vi "ConvertGoop3ToGoop4_CreateInPlacementNode.vi"(8 "error in (no error)":errorcluster, 11 "ViRefIn":refnum<vi>) -> (0 "error out":errorcluster, 3 "ViRefOut":refnum<vi>)   [LabVIEW 2012]
uses:
  <resource>/Framework/Providers/Open_GDS/ClassProviders/Common/ScriptingFunctions/Scripting_FollowWireDownStreams_StopCriteria.ctl
  <resource>/Framework/Providers/Open_GDS/ClassProviders/Common/ScriptingFunctions/Scripting_NodeInfo.ctl
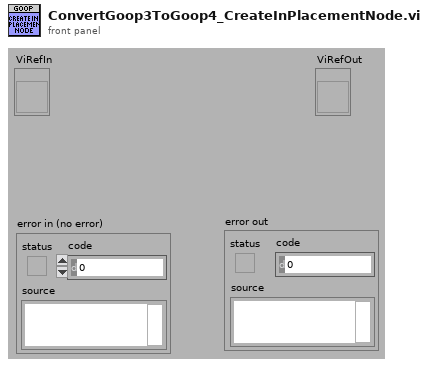
[diagram p1: front panel]
types:
  T1 = typedef "Scripting_FollowWireDownStreams_StopCriteria.ctl" = cluster{"ReachedANyOfTheseNodes":refnum<vi>[], "NodeType":string[], "VINames":string[], "AddTheseNodes":bool, "ALsoSerachOtherDrainNodes":bool}
  T2 = cluster{"Term Refnum Out":refnum<vi>, refnum<vi>[]}[]
  T3 = typedef "Scripting_NodeInfo.ctl" = cluster{"Type":string, "Style":string, "ObjectRef":refnum<vi>, "Terms":refnum<vi>[], "Sources":refnum<vi>[], "Drains":refnum<vi>[], "DrainsSourcesTerms":refnum<vi>[], "SourcesDrainTerms":cluster{"DrainsTerms":refnum<vi>[]}[], "UpperLeftPosition":cluster{"Left":i32, "Top":i32}, "LowerRightPosition":cluster{"Right":i32, "Bottom":i32}}
  T4 = typedef "LVPositionTypeDef.ctl" = cluster{"Left":i32, "Top":i32}
  T5 = typedef "LVBoundsTypeDef.ctl" = cluster{"Width":u32, "Height":u32}
  T6 = cluster{"Term Refnum Out":refnum<vi>, refnum<vi>[]}
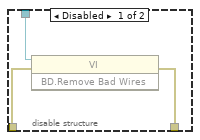
[diagram p2: hidden frame]
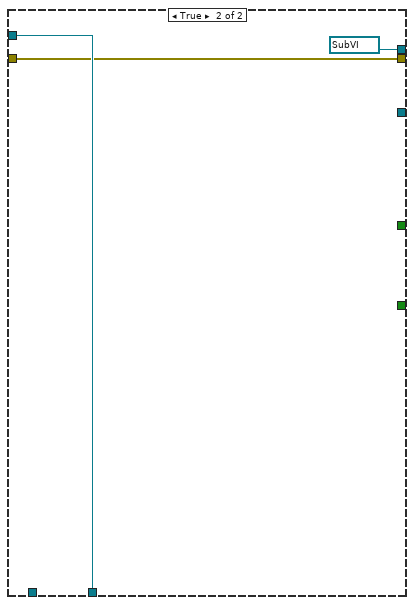
[diagram p5: hidden frame]
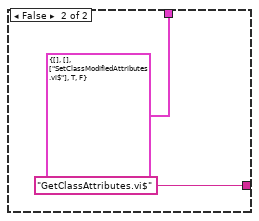
[diagram p7: hidden frame]
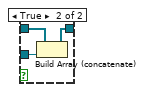
[diagram p11: hidden frame]
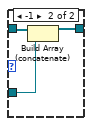
[diagram p12: hidden frame]
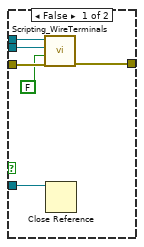
[diagram p15: hidden frame]
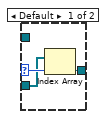
[diagram p19: hidden frame]
diagram:
  # "For every node\nGet all terms\nGet all sources\nGet all drains\nGet all sources drains\nget all drains sources"
  # "Get all nodes:\n-Along the 3 wires\n-All nodes between Get and Set"
  # "Find Get Attribute\nFollow the object wire until we get to the Set Attribute\n-All nodes passed will be inside the IPN\n-Check if there sources are constants and if so, are they inside to the left of GetA\n -For All UnBundler, check if one path leads to one of the Bundler, if so marks all object in that path"
  n1 = case shown="No Error" "error in (no error)" {
    selector: "error in (no error)" -> [w9 w627]
    tunnel: [w7 w627] -> w3
    tunnel: "ViRefIn" -> [w13 _]
    frame No Error {
      w4 = FALSE
      # "C:\\Projects\\GOOP3_To_GOOP4\\BaseSub\\Sub class\\SetClassAttribute.vi"
      n2 = property class="VI"(reference=w13, error in=w9) -> (reference out=w5:refnum<vi>, error out=w14:errorcluster, "Name"=w12:string)
      n3 = Match Pattern(string=w12, regular expression="TP_XA173 WriteConfig.vi") -> (offset past match=w11:i32)  [unwired: 1 in, 3 out]
      n4 = Greater Or Equal To 0?(x=w11) -> ()  [unwired: 1 out]
      n5 = property class="VI"(reference=w5, error in=w14, "BDWin.Open"=w4) -> (error out=w17:errorcluster)  [unwired: 1 out]
      n6 = case shown="True" w4 {
        frame False {
        }
        frame True {
        }
      }
      n7 = call <resource>:"Scripting_FindNodeOnDiagram_1.vi"("ViRef(Ignored If Not Wired)"=w5, "NodeTypesToSearchFor"=string[] ["SubVI"], "error in (no error)"=w17) -> ("Nodes"=w18:refnum<vi>[], "error out"=w19:errorcluster)  [unwired: 15 in]
      n8 = for {
        tunnel: w18 -> [w29] mode=indexing
        shift-right: [w27] -> w8
        shift-left: w19 -> [w43]
        tunnel: w5 -> [w39]
        shift-right: [w32] -> w10
        shift-left: refnum<vi>[] [] -> [w31]
        tunnel: [w30] -> w15 mode=indexing
        tunnel: w5 -> [w25]
        n9 = Not A Number/Path/Refnum?(number/path/refnum=w29) -> (NaN/Path/Refnum?=w28:bool)
        n10 = case shown="False" w28 {
          tunnel: w43 -> [w54 w81]
          tunnel: [w52 refnum<vi> refnum ("WhileLoop")] -> w42
          tunnel: [w51 w81] -> w41
          tunnel: [w50 _] -> w40
          tunnel: [w49 _] -> w35
          tunnel: [w48 _] -> w34
          tunnel: w31 -> [w47 _]
          tunnel: [w45 w82] -> w30
          tunnel: w29 -> [w44 w82]
          frame False {
            n11 = To More Specific Class(target class=refnum<vi> refnum ("WhileLoop"), reference=w44, error in=w54) -> (specific class reference=w45:refnum<vi>, error out=w53:errorcluster)
            n12 = Search 1D Array(1D array=w47, element=w45) -> (index of element=w46:i32)  [unwired: 1 in]
            n13 = case shown="-1" w46 {
              tunnel: w53 -> [w56 w79]
              tunnel: [w57 w77] -> w52
              tunnel: [w56 w76] -> w51
              tunnel: [_ w75] -> w50
              tunnel: [_ w60] -> w49
              tunnel: [_ w59] -> w48
              tunnel: w45 -> [w57 w58]
              frame 0, Default {
                # "It has already been deleted"
              }
              frame -1 {
                n14 = property class="SubVI"(reference=w58, error in=w79) -> (reference out=w77:refnum<vi>, error out=w76:errorcluster, "VIName"=w63:string, "Owner"=w75:refnum<vi>, "Desc"=w62:string)
                n15 = Match Pattern(string=w62, regular expression="M\\[[0-9]+:[0-9]+\\]") -> (offset past match=w72:i32)  [unwired: 1 in, 3 out]
                n16 = Match Pattern(string=w62, regular expression="CM\\[[0-9]+:[0-9]+\\]") -> (offset past match=w67:i32)  [unwired: 1 in, 3 out]
                n17 = Match Pattern(string=w63, regular expression="GetAttributes.vi$") -> (offset past match=w73:i32)  [unwired: 1 in, 3 out]
                n18 = Match Pattern(string=w63, regular expression="GetClassAttributes.vi$") -> (offset past match=w66:i32)  [unwired: 1 in, 3 out]
                n19 = Greater Or Equal To 0?(x=w72) -> (x >= 0?=w70:bool)
                n20 = Greater Or Equal To 0?(x=w67) -> (x >= 0?=w69:bool)
                n21 = Greater Or Equal To 0?(x=w73) -> (x >= 0?=w71:bool)
                n22 = Greater Or Equal To 0?(x=w66) -> (x >= 0?=w68:bool)
                n23 = And(x=w71, y=w70) -> (x .and. y?=w59:bool)
                n24 = And(x=w68, y=w69) -> (x .and. y?=w61:bool)
                n25 = Or(x=w59, y=w61) -> (x .or. y?=w60:bool)
              }
            }
          }
          frame True {
          }
        }
        n26 = case shown="True" w35 {
          tunnel: w42 -> [w119 _]
          tunnel: w41 -> [w121 w626]
          tunnel: [w92 w626] -> w27
          tunnel: w40 -> [w112 _]
          tunnel: w39 -> [w85 _]
          tunnel: [w106 _] -> w38
          tunnel: [w101 _] -> w37
          tunnel: [w100 _] -> w36
          tunnel: w34 -> [w98 _]
          tunnel: [w95 _] -> w33
          tunnel: [w94 w625] -> w32
          tunnel: w31 -> [w93 w625]
          tunnel: [w86 _] -> w26
          tunnel: w25 -> [w84 _]
          frame True {
            # "All Get Att Drains\n(Left Terminals)"
            # "ErrorOut"
            # "Att"
            # "ErrorOut"
            # "Att"
            n27 = property class="SubVI"(reference=w119, error in=w121) -> (reference out=w111:refnum<vi>, error out=w118:errorcluster, "Terms[]"=w89:refnum<vi>[])
            n28 = call <resource>:"Scripting_SortTerminals.vi"("Terminals[]"=w89) -> ("TerminalsOut[]"=w83:refnum<vi>[])  [unwired: 8 in, 2 out]
            n29 = Array Size(array=w89) -> (size(s)=w122:i32)
            n30 = case shown="True" w98 {
              tunnel: [T1 {"ReachedANyOfTheseNodes"=[], "NodeType"=[], "VINames"=["SetModifiedAttributes.vi$"], "AddTheseNodes"=TRUE, "ALsoSerachOtherDrainNodes"=FALSE} ("StopCriteria") T1 {"ReachedANyOfTheseNodes"=[], "NodeType"=[], "VINames"=["SetClassModifiedAttributes.vi$"], "AddTheseNodes"=TRUE, "ALsoSerachOtherDrainNodes"=FALSE} ("StopCriteria")] -> w97
              tunnel: ["GetAttributes.vi$" ("regular expression") "GetClassAttributes.vi$" ("regular expression")] -> w96
              frame True {
              }
              frame False {
              }
            }
            n31 = for {
              tunnel: w89 -> [w130] mode=indexing
              shift-right: [w127] -> w87
              shift-left: refnum<vi>[] [] -> [w128]
              n32 = property class="Term"(reference=w130) -> (reference out=w129:refnum<vi>, "IsSource"=w126:bool, "Wire"=w123:refnum<vi>)  [unwired: 1 in, 1 out]
              n33 = Not A Number/Path/Refnum?(number/path/refnum=w123) -> (NaN/Path/Refnum?=w125:bool)
              n34 = Compound Arithmetic op=AND(w126, invert w125) -> (w124:bool)
              n35 = case shown="False" w124 {
                tunnel: w129 -> [w133 _]
                tunnel: w128 -> [w132 w134]
                tunnel: [w131 w134] -> w127
                frame False {
                  n36 = Build Array (concatenate)(w132, w133) -> (w131:refnum<vi>[])
                }
                frame True {
                }
              }
              n37 = Close Reference(reference=w123) -> ()  [unwired: 1 in, 1 out]
            }
            n38 = case shown="20" w122 {
              tunnel: [9 ("index") 15 ("index")] -> w104
              tunnel: [8 ("index") 14 ("index")] -> w103
              tunnel: [11 ("index") 19 ("index")] -> w105
              tunnel: [10 ("index") 17 ("index")] -> w102
              tunnel: [1 ("index") 2 ("index")] -> w90
              frame 12, Default {
              }
              frame 20 {
              }
            }
            n39 = Index Array(array=w83, index #1=w105, index #2=w104, index #3=w103, index #4=w102) -> (element #1=w114:refnum<vi>, element #2=w120:refnum<vi>, element #3=w117:refnum<vi>, element #4=w108:refnum<vi>)
            n40 = call <resource>:"Scripting_FollowWireDownStreams.vi"("Term Refnum"=w117, "NodeTypesToFind"=string[] ["SubVI"] ("NodeTypesToSearchFor"), "error in"=w118, "MainitainDataType"=TRUE ("MainitainDateType(True)"), "StopCriteria"=w97) -> ("Nodes"=w106:refnum<vi>[], "error out"=w109:errorcluster)  [unwired: 11 in, 2 out]
            n41 = Array Size(array=w106) -> (size(s)=w115:i32)
            n42 = Delete From Array(array=w106) -> (deleted portion=w113:refnum<vi>, array with subset deleted=w107:refnum<vi>[])  [unwired: 2 in]
            n43 = case shown="1.." w115 {
              tunnel: w120 -> [_ w219]
              tunnel: w114 -> [_ _]
              tunnel: w113 -> [_ w237]
              tunnel: w112 -> [_ w230]
              tunnel: w111 -> [_ w155]
              tunnel: [w140 w142] -> w110
              tunnel: w109 -> [w140 w148]
              tunnel: w108 -> [_ w208]
              tunnel: w90 -> [_ w223]
              tunnel: w107 -> [_ w220]
              tunnel: w105 -> [_ w146]
              tunnel: w104 -> [_ w218]
              tunnel: w103 -> [_ w217]
              tunnel: w102 -> [_ w216]
              tunnel: [_ w215] -> w101
              tunnel: [_ w214] -> w100
              tunnel: w85 -> [_ w165]
              tunnel: w96 -> [_ w191]
              tunnel: [_ w178] -> w95
              tunnel: [w139 w176] -> w94
              tunnel: w93 -> [w139 w175]
              tunnel: [_ w159] -> w91
              tunnel: w87 -> [_ w156]
              tunnel: [_ w151] -> w86
              tunnel: w84 -> [_ w149]
              tunnel: w83 -> [_ w147]
              frame 0, Default {
                # "We can't find the SetModifyVI, something is wrong"
              }
              frame 1.. {
                (unwired) refnum<vi> refnum ("element")
                w193 = refnum<vi>[] []
                w234 = refnum<vi> refnum  # InPlaceElementStructure
                w235 = 2360 items=[".NET Container"=2125, ".NET Refnum"=3441, "2D Picture"=3508, "3D Picture"=23776, "Absolute Value"=1054, "Access Rights"=1412, "ActiveX Container"=2072, "Add"=3915, "Add 1"=1050, "Add Array Elements"=1903, "Agitator"=3831, "AllSpoll"=1960, "Always Copy"=2400, "And"=1061, "And Array Elements"=1911, "Append True/False String"=1511, "Application Refnum"=3412, "Array"=21608, "Array 1"=3300, "Array Constant"=2070, "Array Interface Control"=23777, "Array Max & Min"=1907, "Array Size"=1809, "Array Subset"=2044, "Array To Cluster"=1168, "Array To Spreadsheet String"=1540, "Array of Strings to Path"=1422, "Atmospheric Tank"=3070, "Atmospheric Tank 1"=21751, "Automation Close"=8001, "Automation Open"=8000, "Automation Refnum"=3410, "Avogadro Constant (1/mol)"=23520, "Base 10 Logarithm Of e"=23512, "Bin"=3073, "Bin 1"=21755, "Bitpack to Array"=3135, "Blocking Variable Read"=23786, "Blocking Variable Write"=23789, "Bluetooth Close Connection"=9148, "Bluetooth Create Listener"=9151, "Bluetooth Discover"=9152, "Bluetooth Network Connection Refnum"=3468, "Bluetooth Open Connection"=9153, "Bluetooth Read"=9149, "Bluetooth Wait On Listener"=9147, "Bluetooth Write"=9150, "Boolean Array To Number"=1815, "Boolean To (0,1)"=1167, "Build Array"=2041, "Build Cluster Array"=2047, "Build Matrix"=8500, "Build Path"=1419, "Build Waveform"=2066, "Bundle"=2049, "Bundle By Name"=2057, "Byte Array To String"=1609, "Byte Stream File Refnum"=3408, "CAN Channel"=21966, "CAN Channel 1"=3340, "CAN Channel 2"=2124, "CAN Channel 3"=21817, "CAN Interface"=3339, "CAN Interface 1"=21815, "CAN Interface 2"=2123, "CAN Interface 3"=21964, "CAN Task"=3470, "CAN Task 1"=3471, "CAN Task 2"=21963, "CAN Task 3"=21789, "CPU Information"=24130, "Call By Reference Node"=3901, "Call Chain"=1999, "Call Library Function Node"=2062, "Call Parent Method"=2354, "Cancel Button"=21739, "Cancel Notification"=9107, "Carriage Return Constant"=23500, "Case Structure"=2001, "Cast Unit Bases"=1079, "Check Valve"=3833, "Checkbox"=3117, "Class Specifier Constant"=2094, "Classic Radio Buttons"=22003, "Clear Fixed-Point Overflow Status"=5562, "Close File"=1405, "Close File 1"=8052, "Close Reference"=8011, "Close Variable Connection"=23783, "Cluster"=3400, "Cluster 1"=21607, "Cluster Constant"=2071, "Cluster To Array"=1169, "Code Interface Node"=2050, "Coerce To Type"=2402, "Color Box"=3013, "Color Box Constant"=2120, "Color Box Thin Border"=2905, "Color Ramp"=3022, "Combo Box"=21604, "Combo Box 1"=3304, "Combo Box Constant"=2088, "Complex Conjugate"=1048, "Complex To Polar"=1045, "Complex To Re/Im"=1044, "Compound Arithmetic"=2200, "Compressor"=3832, "Concatenate Strings"=2040, "Conditional Disable Structure"=2064, "Constructor Node"=3904, "Control & Simulation Loop"=2099, "Control Help Window"=1353, "Control Online Help"=1355, "Control Refnum"=3419, "Convert Unit"=2059, "Conveyer"=3827, "Copy"=1416, "Copy 1"=8053, "Cosecant"=1204, "Cosine"=1201, "Cotangent"=1205, "Create Folder"=8055, "Create User Event"=2073, "Current Processor ID"=24131, "Current VI's Menubar"=9000, "Current VI's Path"=1426, "DAQmx Analog Trigger Source"=3336, "DAQmx Analog Trigger Source 1"=2119, "DAQmx Analog Trigger Source 2"=21951, "DAQmx Analog Trigger Source 3"=21774, "DAQmx Device Name"=21773, "DAQmx Device Name 1"=21950, "DAQmx Device Name 2"=2093, "DAQmx Device Name 3"=3318, "DAQmx Global Channel"=3443, "DAQmx Global Channel 1"=21770, "DAQmx Global Channel 2"=21957, "DAQmx Global Channel 3"=3430, "DAQmx Physical Channel"=3335, "DAQmx Physical Channel 1"=21954, "DAQmx Physical Channel 2"=2118, "DAQmx Physical Channel 3"=21777, "DAQmx Scale Name"=21952, "DAQmx Scale Name 1"=21775, "DAQmx Scale Name 2"=3317, "DAQmx Scale Name 3"=2116, "DAQmx Switch"=21953, "DAQmx Switch 1"=3337, "DAQmx Switch 2"=2121, "DAQmx Switch 3"=21776, "DAQmx Task Name"=3442, "DAQmx Task Name 1"=3434, "DAQmx Task Name 2"=21959, "DAQmx Task Name 3"=21778, "DAQmx Terminal"=21955, "DAQmx Terminal 1"=2117, "DAQmx Terminal 2"=21781, "DAQmx Terminal 3"=3319, "Data Cache Size"=24132, "Data Log File Refnum"=3402, "DataSocket Close"=1085, "DataSocket Open"=1084, "DataSocket Read"=1086, "DataSocket Refnum"=3417, "DataSocket Write"=1087, "Date/Time To Seconds"=1308, "Decimal Digit?"=1119, "Decimal String To Number"=1184, "Decimate 1D Array"=2046, "DecomposeArray"=2412, "DecomposeLockDataValRef"=2406, "DecomposeVariant"=2404, "Decrement"=1058, "Default Directory"=1427, "Delete"=8056, "Delete 1"=1417, "Delete Data Value Reference"=2409, "Delete From Array"=3912, "Delete Menu Items"=9004, "Delete Variant Attribute"=8206, "Delete Waveform Attribute"=8209, "Deny Access"=8057, "Dequeue Element"=9113, "Destroy User Event"=2075, "DevClear"=1961, "DevClearList"=1962, "Device Control/Status"=1433, "Device Refnum"=3405, "Diagram Disable Structure"=2054, "Dial"=3050, "Dial 1"=21732, "Digital Data"=3210, "Digital Data 1"=21216, "Digital Waveform Graph"=21718, "Digital Waveform Graph 1"=3511, "Direct Variable Read"=23785, "Direct Variable Write"=23788, "Divide"=1053, "Divide 1"=3918, "Dlg CheckBox"=21924, "Dlg Horiz Scrollbar"=21905, "Dlg Numeric"=2100, "Dlg Numeric 2"=3006, "Dlg String"=2110, "Dlg Vert Scrollbar"=21906, "Down Arrow"=3824, "Down Bow Valve"=3707, "Down Bow Valve 1"=21767, "Down Bow Valve 2"=3807, "Down Rect Valve"=21766, "Down Rect Valve 1"=3706, "Down Rect Valve 2"=3806, "Down Tee"=3818, "Down Tee 1"=3718, "EOF"=1410, "Elementary Charge (C)"=23517, "Empty Array?"=23063, "Empty Path Constant"=23523, "Empty String Constant"=23503, "Empty String/Path?"=1112, "Enable Menu Tracking"=9002, "EnableLocal"=1963, "EnableRemote"=1964, "End of Line Constant"=23525, "Enqueue Element"=9111, "Enqueue Element At Opposite End"=9129, "Enum"=3023, "Enum 1"=21605, "Enum Constant"=2090, "Equal To 0?"=1113, "Equal?"=1102, "Error Ring Constant"=2039, "Event Callback Refnum"=3435, "Event Data Node"=2102, "Event Structure"=2052, "Exchanger"=3828, "Exclusive Or"=1063, "Exponential"=1211, "Exponential (Arg) -1"=1222, "Expression Node"=2201, "FIFO Refnum"=3474, "False Constant"=2006, "Feedback Node, Feedback Node 1"=2353, "FieldPoint IO Point"=21784, "FieldPoint IO Point 1"=3440, "FieldPoint IO Point 2"=3439, "File Dialog"=8058, "File Dialog 1"=8081, "File Path Control"=21730, "File Path Control 1"=3203, "File Path Indicator"=21731, "File Path Indicator 1"=3204, "File/Directory Info"=1413, "File/Directory Info 1"=8082, "FindLstn"=1965, "FindRQS"=1966, "First Call?"=1083, "Fixed-Point Overflow?"=5565, "Fixed-Point to Integer Cast"=5566, "Flat Box"=3602, "Flat Circle"=3605, "Flat Down Triangle"=3623, "Flat Frame"=3608, "Flat Left Triangle"=3620, "Flat Right Triangle"=3621, "Flat Round Button"=3102, "Flat Rounded Box"=3611, "Flat Sequence Structure"=2069, "Flat Square Button"=3103, "Flat Up Triangle"=3622, "Flatten To String"=1164, "Flatten To XML"=8400, "Flattened String To Variant"=8202, "Floating Point Equal?"=23064, "Flush File"=8059, "Flush File 1"=1406, "Flush Queue"=9114, "For Loop"=2002, "Fork"=2194, "Format Date/Time String"=8100, "Format Into File"=2083, "Format Into String"=2081, "Format Value"=1512, "Formula Node"=2004, "Fract/Exp String To Number"=1187, "Framed Color Box"=21019, "Framed Color Box 1"=3008, "Free Label"=2321, "Furnace"=3829, "GPIB Clear"=1954, "GPIB Initialization"=1957, "GPIB Misc"=1956, "GPIB Read"=1951, "GPIB Serial Poll"=1955, "GPIB Status"=1959, "GPIB Trigger"=1953, "GPIB Wait"=1958, "GPIB Write"=1950, "Gauge"=21009, "Gauge 1"=3040, "Generate Front Panel Activity"=1329, "Generate Occurrence"=1700, "Generate User Event"=2074, "Generate User-Defined Trace Event"=2250, "Get Datalog Position"=8061, "Get Date/Time In Seconds"=1303, "Get Date/Time String"=1600, "Get Drag Drop Data"=9154, "Get File Position"=8062, "Get File Size"=8063, "Get Fixed-Point Components"=11163, "Get Help Window Status"=1354, "Get Matrix Diagonal"=8501, "Get Matrix Elements"=8502, "Get Menu Item Info"=9005, "Get Menu Selection"=9001, "Get Menu Short Cut Info"=9007, "Get Notifier Status"=9103, "Get Number of Records"=8064, "Get Permissions"=8065, "Get Queue Status"=9110, "Get Submatrix"=8503, "Get Type and Creator"=8066, "Get Variant Attribute"=8205, "Get Volume Info"=8067, "Get Waveform Attribute"=8208, "Get Waveform Components"=2067, "Global Variable"=2060, "Gravitational Constant (N m2/kg2)"=23519, "Greater Or Equal To 0?"=1114, "Greater Or Equal?"=1103, "Greater Than 0?"=1117, "Greater?"=1110, "Handle Peek"=1604, "Handle Poke"=1605, "Hex Digit?"=1123, "Hexadecimal String To Number"=1185, "Hopper"=21754, "Hopper 1"=3072, "Horiz Line"=3821, "Horiz Pipe"=3710, "Horiz Pipe 1"=3810, "Horizontal Button Box"=3636, "Horizontal Fill Slide"=3012, "Horizontal Fill Slide 1"=21100, "Horizontal Graduated Bar"=21106, "Horizontal Pointer Slide"=21101, "Horizontal Pointer Slide 1"=3011, "Horizontal Progress Bar"=21102, "Horizontal Scrollbar"=21110, "Horizontal Slide"=3010, "Horizontal Slide Switch"=3114, "Horizontal Smooth Box"=3633, "Horizontal Splitter Bar"=21861, "Horizontal Splitter Bar (Classic)"=21863, "Horizontal Splitter Bar (System)"=21865, "Horizontal Switch"=3108, "Horizontal Tank"=3071, "Horizontal Toggle Switch"=3110, "Horizontal Toggle Switch 1"=21700, "Hyperbolic Cosecant"=23053, "Hyperbolic Cosine"=1215, "Hyperbolic Cotangent"=23055, "Hyperbolic Secant"=23054, "Hyperbolic Sine"=1214, "Hyperbolic Tangent"=1216, "IMAQ Session"=3415, "IP To String"=1710, "IVI Delete Session"=8103, "IVI Logical Name"=3420, "IVI Logical Name 1"=3414, "IVI Logical Name 2"=21736, "IVI New Session"=8102, "Implies"=1080, "In Place Element Structure"=2360, "In Range and Coerce"=1127, "Include Fixed-Point Overflow Status"=5564, "Increment"=1057, "Index & Bundle Cluster Array"=2056, "Index Array"=2042, "Index String Array"=1531, "Initialize Array"=2053, "Inline C Node"=2104, "Insert Into Array"=3911, "Insert Menu Items"=9003, "Integer to Fixed-Point Cast"=5567, "Intensity Chart"=21719, "Intensity Chart 1"=3509, "Intensity Graph"=21720, "Intensity Graph 1"=3510, "Interleave 1D Arrays"=2045, "Interpolate 1D Array"=1905, "Inverse Cosecant"=23050, "Inverse Cosine"=1207, "Inverse Cotangent"=23052, "Inverse Hyperbolic Cosecant"=23056, "Inverse Hyperbolic Cosine"=1218, "Inverse Hyperbolic Cotangent"=23058, "Inverse Hyperbolic Secant"=23057, "Inverse Hyperbolic Sine"=1217, "Inverse Hyperbolic Tangent"=1219, "Inverse Secant"=23051, "Inverse Sine"=1206, "Inverse Tangent"=1208, "Inverse Tangent (2 Input)"=1228, "Invoke Node"=3900, "IrDA Close Connection"=9144, "IrDA Create Listener"=9140, "IrDA Discover"=9141, "IrDA Network Connection Refnum"=3450, "IrDA Open Connection"=9142, "IrDA Read"=9145, "IrDA Wait On Listener"=9143, "IrDA Write"=9146, "Join"=2195, "Join Numbers"=1171, "Junction"=2197, "Knob"=21000, "Knob 1"=3005, "LED Button"=3116, "LabVIEW Object"=3457, "Label"=21960, "Labeled Oblong Button"=3125, "Labeled Rectangular Button"=3124, "Labeled Round Button"=3122, "Labeled Square Button"=3123, "Leak Variant Value Reference"=2410, "Left Arrow"=3826, "Left Bow Valve"=3701, "Left Bow Valve 1"=3801, "Left Bow Valve 2"=21761, "Left Down Elbow"=3711, "Left Down Elbow 1"=3811, "Left Pump"=3713, "Left Pump 1"=3813, "Left Rect Valve"=3700, "Left Rect Valve 1"=21760, "Left Rect Valve 2"=3800, "Left Tee"=3709, "Left Tee 1"=3809, "Left Up Elbow"=3808, "Left Up Elbow 1"=3708, "Less Or Equal To 0?"=1115, "Less Or Equal?"=1104, "Less Than 0?"=1118, "Less?"=1111, "Lexical Class"=1126, "Line Feed Constant"=23501, "List Directory"=1418, "List Folder"=8083, "Listbox"=21792, "Listbox 1"=21806, "Listbox Symbol Ring Constant"=2038, "Local Variable"=2061, "Lock Range"=1411, "Logarithm Base 10"=1210, "Logarithm Base 2"=1225, "Logarithm Base X"=1224, "Logical Shift"=1081, "Lossy Enqueue Element"=9130, "Lowered Rounded Box"=3638, "MATLAB script"=9020, "Machine Epsilon"=23528, "MakeAddr"=1967, "Mantissa & Exponent"=1150, "Match First String"=1532, "Match Pattern"=1535, "Match True/False String"=1533, "MathScript Call By Reference Node"=3906, "MathScript Node"=2357, "Matrix Size"=8507, "Max & Min"=1108, "Menu Refnum"=3413, "Menu Ring"=3018, "Menu Ring 1"=21600, "Menu-Popup Ring"=3017, "Merge Signals"=2350, "Meter"=21008, "Meter 1"=3030, "Mixed Signal Graph"=21721, "Molar Gas Constant (J/(mol K))"=23522, "Motion Resource"=21787, "Motion Resource 1"=3448, "Motion Resource 2"=3449, "Motor"=3720, "Motor 1"=3820, "Move"=1415, "Move 1"=8068, "Multi-Segment Pipe"=23780, "Multicolumn Listbox"=21799, "Multicolumn Listbox 1"=21791, "Multiple Selection Listbox"=3208, "Multiply"=1052, "Multiply 1"=3917, "Multiply Array Elements"=1904, "Multirate Structure"=2199, "Natural Logarithm"=1209, "Natural Logarithm (Arg +1)"=1221, "Natural Logarithm Base"=23510, "Natural Logarithm Of 10"=23513, "Natural Logarithm Of 2"=23514, "Natural Logarithm Of Pi"=23508, "Negate"=1069, "Negative Infinity"=23509, "New Data Value Reference"=2408, "New Directory"=1402, "New File"=1404, "New VI"=8014, "New VI Object"=8015, "Not"=1064, "Not A Number/Path/Refnum?"=1128, "Not A Path Constant"=23524, "Not And"=1071, "Not Equal To 0?"=1116, "Not Equal?"=1105, "Not Exclusive Or"=1073, "Not Or"=1072, "Not a Refnum Constant"=23526, "Not a Shared Variable"=23527, "Notifier Refnum"=3423, "Number To Boolean Array"=1814, "Number To Decimal String"=1180, "Number To Engineering String"=1183, "Number To Exponential String"=1505, "Number To Fractional String"=1506, "Number To Hexadecimal String"=1181, "Number To Octal String"=1182, "Number of Cache Levels"=24133, "Numeric Constant"=2005, "Numeric Control"=3000, "Numeric Control 1"=21003, "Numeric Indicator"=3001, "Numeric Indicator 1"=21004, "OK Button"=21738, "OLE Variant"=3150, "Obtain Notifier"=9101, "Obtain Queue"=9108, "Occurrence Refnum"=3406, "Octal Digit?"=1129, "Octal String To Number"=1186, "Old VISA Open"=1921, "One Button Dialog"=1340, "Open Application Reference"=8012, "Open Device"=1430, "Open File"=1403, "Open Tank"=21752, "Open Tank 1"=3074, "Open VI Object Reference"=8013, "Open VI Reference"=8010, "Open Variable Connection"=23779, "Open Variable Connection in Background"=23791, "Open and Verify Variable Connection"=23790, "Open/Create/Replace Datalog"=8054, "Open/Create/Replace File"=8050, "Or"=1062, "Or Array Elements"=1910, "PPoll"=1969, "PPollConfig"=1970, "PPollUnconfig"=1971, "Package Matrix"=23001, "PassControl"=1968, "Path Constant"=2009, "Path To String"=1077, "Path Type"=1421, "Path to Array of Strings"=1423, "Pi"=23504, "Pi Divided By 2"=23506, "Pi Multiplied By 2"=23505, "Pick Line"=1510, "Pict Ring"=21602, "Pict Ring 1"=3015, "PixMap"=3505, "PixMap (Do not touch it!!)"=3507, "Planck's Constant (J/Hz)"=23516, "Platform Flat Square Button"=3134, "Plug-In Control"=21820, "Polar To Complex"=1047, "Polar To Re/Im"=23061, "Positive Infinity"=23515, "Power Of 10"=1212, "Power Of 2"=1223, "Power Of X"=1213, "Preserve Run-Time Class"=8018, "Pressure Tank"=3075, "Pressure Tank 1"=21753, "Preview Queue Element"=9112, "Printable?"=1124, "Property Node"=1920, "Pulldown Menu Ring"=3061, "Push Button"=21001, "Queue Refnum"=3424, "Quit LabVIEW"=1352, "Quotient & Remainder"=1056, "RT FIFO Create"=24000, "RT FIFO Delete"=24003, "RT FIFO Read"=24001, "RT FIFO Write"=24002, "Radio Buttons"=22001, "Raised Box"=3600, "Raised Box 1"=3637, "Raised Circle"=3603, "Raised Down Triangle"=3615, "Raised Frame"=3606, "Raised Left Triangle"=3612, "Raised Right Triangle"=3613, "Raised Rounded Box"=3609, "Raised Up Triangle"=3614, "Random Number (0-1)"=1070, "RcvRespMsg"=1972, "Re/Im To Complex"=1046, "Re/Im To Polar"=23060, "Read Datalog"=8069, "Read Device"=1432, "Read File"=1407, "Read Variable"=23781, "Read from Binary File"=8051, "Read from Text File"=8070, "ReadStatus"=1973, "Receive"=1974, "ReceiveSetup"=1975, "Recessed Box"=3601, "Recessed Circle"=3604, "Recessed Down Triangle"=3619, "Recessed Frame"=3607, "Recessed Left Triangle"=3616, "Recessed Menu Ring"=3019, "Recessed Right Triangle"=3617, "Recessed Rounded Box"=3610, "Recessed Up Triangle"=3618, "Reciprocal"=1059, "Reciprocal Of Pi"=23507, "Reciprocal Of e"=23511, "RecomposeArray"=2403, "RecomposeUnlockDataValRef"=2407, "RecomposeVariant"=2405, "Rectangular Stop Button"=3128, "Refnum to Path"=1424, "Refnum to Session"=2306, "Region"=2196, "Register Event Callback"=2078, "Register For Events"=2065, "Register Session"=2319, "Release Notifier"=9102, "Release Queue"=9109, "Remove Fixed-Point Overflow Status"=5563, "Replace Array Subset"=3910, "Replace Substring"=3913, "Request Deallocation"=1610, "ResetSys"=1976, "Reshape Array"=2055, "Resize Matrix"=8508, "Reverse 1D Array"=1900, "Reverse String"=1537, "Right Arrow"=3825, "Right Bow Valve"=21765, "Right Bow Valve 1"=3705, "Right Bow Valve 2"=3805, "Right Down Elbow"=3817, "Right Down Elbow 1"=3717, "Right Pump"=3719, "Right Pump 1"=3819, "Right Rect Valve"=3804, "Right Rect Valve 1"=3704, "Right Rect Valve 2"=21764, "Right Tee"=3715, "Right Tee 1"=3815, "Right Up Elbow"=3814, "Right Up Elbow 1"=3714, "Ring Constant"=2008, "Rocker"=21002, "Rotary Feeder"=3830, "Rotate"=1082, "Rotate 1D Array"=1906, "Rotate Left With Carry"=1606, "Rotate Right With Carry"=1607, "Rotate String"=1536, "Round Button"=3100, "Round LED"=3120, "Round LED 1"=21012, "Round Light"=3104, "Round Push Button"=3112, "Round Push Button 2"=3118, "Round Radio Button"=3106, "Round Stop Button"=3127, "Round To Nearest"=1055, "Round Toward +Infinity"=1076, "Round Toward -Infinity"=1075, "Rydberg Constant (1/m)"=23521, "Scale By Power Of 2"=1074, "Scan From File"=2082, "Scan From String"=2080, "Scan String For Tokens"=8101, "Scan Value"=1534, "Scanned Variable Read"=23784, "Scanned Variable Write"=23787, "Search 1D Array"=1901, "Search and Replace String"=3914, "Search/Split String"=1538, "Secant"=1203, "Seconds To Date/Time"=1309, "Seek"=1409, "Select"=1516, "Send"=1977, "Send Notification"=9104, "SendCmds"=1978, "SendDataBytes"=1979, "SendIFC"=1980, "SendLLO"=1982, "SendList"=1981, "SendSetup"=1983, "Session to Refnum"=2307, "Set Datalog Position"=8072, "Set File Position"=8073, "Set File Size"=8074, "Set Matrix Diagonal"=8504, "Set Matrix Elements"=8505, "Set Menu Item Info"=9006, "Set Number of Records"=8075, "Set Occurrence"=1702, "Set Permissions"=8076, "Set Submatrix"=8506, "Set Type and Creator"=8077, "Set Variant Attribute"=8204, "Set Waveform Attribute"=8207, "SetRWLS"=1984, "SetTimeOut"=1985, "Shared Variable"=23778, "Shared Variable Constant"=3473, "Shared Variable Control"=3472, "Shared Variable Control 1"=21814, "Shared Variable to String"=1831, "Sign"=1049, "Simple Horizontal Slide"=3003, "Simple Numeric"=3029, "Simple Numeric 1"=2900, "Simple String"=2115, "Simple Vertical Slide"=3002, "Sinc"=1227, "Sine"=1200, "Sine & Cosine"=1220, "Size Handle"=1603, "Slide Switch"=21011, "Sort 1D Array"=1120, "Sort Array of String, Sort Array of String 1"=23065, "Speed Of Light In Vacuum (m/sec)"=23518, "Split 1D Array"=1908, "Split Button"=21020, "Split Number"=1170, "Split Signals"=2351, "Spreadsheet String To Array"=1539, "Square"=23059, "Square Button"=3101, "Square LED"=3121, "Square LED 1"=21013, "Square Light"=3105, "Square Push Button"=3113, "Square Push Button 2"=3119, "Square Radio Button"=3107, "Square Root"=1060, "Stacked Sequence Structure"=2000, "State"=2198, "State Diagram"=2051, "Static VI Reference"=2084, "Stop"=1350, "Stop Button"=21230, "String Constant"=2007, "String Control"=3200, "String Control 1"=21701, "String Indicator"=3201, "String Indicator 1"=21702, "String Length"=1502, "String Subset"=1503, "String To Byte Array"=1608, "String To IP"=1711, "String To Path"=1078, "String to Shared Variable"=1830, "Strip Path"=1420, "SubPanel"=21810, "SubPanel (Classic)"=21811, "SubPanel (System)"=21823, "Subtract"=1051, "Subtract 1"=3916, "Swap Bytes"=1162, "Swap Values"=2401, "Swap Vector Element"=1912, "Swap Words"=1163, "System Button"=3130, "System Cancel Button"=3131, "System Checkbox"=3132, "System Chiseled Line"=3632, "System Colored Rectangle"=3625, "System Combo Box"=21917, "System Enum"=3062, "System Horizontal Pointer Slide"=21902, "System Horizontal Progress Bar"=21910, "System Horizontal Slide"=21904, "System Label"=21961, "System Listbox"=21805, "System Mixed Checkbox"=21333, "System Multicolumn Listbox"=21798, "System Numeric"=21919, "System Path Control"=21922, "System Pict Ring"=21925, "System Radio Button"=3133, "System Radio Buttons"=22002, "System Recessed Frame"=3624, "System Ring"=3060, "System Spin Control"=21900, "System String"=21920, "System Tab Control"=3331, "System Table"=21797, "System Time Stamp"=21967, "System Tree"=21794, "System Vertical Pointer Slide"=21901, "System Vertical Progress Bar"=21909, "System Vertical Slide"=21903, "TCP Close Connection"=1713, "TCP Create Listener"=1717, "TCP Flattened Read"=1718, "TCP Flattened Write"=1719, "TCP Flex Read"=1720, "TCP Flex Write"=1721, "TCP Network Connection Refnum"=3407, "TCP Open Connection"=1715, "TCP Read"=1716, "TCP Wait On Listener"=1712, "TCP Write"=1714, "TDMS Close"=24113, "TDMS Defragment"=24119, "TDMS File"=3477, "TDMS Flush"=24117, "TDMS Get Properties"=24115, "TDMS List Contents"=24116, "TDMS Open"=24112, "TDMS Read"=24111, "TDMS Refnum To File ID"=24120, "TDMS Set Properties"=24114, "TDMS Write"=24110, "TDMS Write IP"=24118, "Tab Constant"=23502, "Tab Control"=3330, "Tab Control 1"=3332, "Table"=21796, "Table 1"=21790, "Tag Attribute Ring"=2063, "Tangent"=1202, "Tank"=21006, "Tank 1"=3020, "Temporary Directory"=1435, "TestSRQ"=1986, "TestSys"=1987, "Text & Pict Ring"=21603, "Text & Pict Ring 1"=3016, "Text Button"=21015, "Text Ring"=21601, "Text Ring 1"=3014, "Text to UTF-8"=23066, "Thermometer"=21007, "Thermometer 1"=3021, "Thick Chiseled Line"=3630, "Thick Line"=3629, "Thick Line with Arrow"=3631, "Thick Lowered Box"=3635, "Thin Chiseled Line"=3627, "Thin Line"=3626, "Thin Line with Arrow"=3628, "Threshold 1D Array"=1909, "Tick Count (ms)"=1300, "Time Stamp Constant"=2068, "Time Stamp Control"=21913, "Time Stamp Control 1"=5555, "Time Stamp Indicator"=21914, "Time Stamp Indicator 1"=5556, "Timed Loop"=5570, "Timed Sequence"=5573, "To Byte Integer"=1140, "To Double Precision Complex"=1152, "To Double Precision Float"=1147, "To Extended Precision Complex"=1154, "To Extended Precision Float"=1149, "To Fixed-Point"=5561, "To Long Integer"=1142, "To Lower Case"=1189, "To More Generic Class"=8017, "To More Specific Class"=8016, "To OLE Variant"=8002, "To Probe String"=2413, "To Quad Integer"=1155, "To Single Precision Complex"=1151, "To Single Precision Float"=1146, "To Time Stamp"=5560, "To Unsigned Byte Integer"=1143, "To Unsigned Long Integer"=1145, "To Unsigned Quad Integer"=1156, "To Unsigned Word Integer"=1144, "To Upper Case"=1188, "To Variant"=8201, "To Word Integer"=1141, "Traditional DAQ Channel"=21733, "Traditional DAQ Channel 1"=2085, "Traditional DAQ Channel 2"=3320, "Transpose 1D Array"=23068, "Transpose 2D Array"=1902, "Transpose Matrix"=8509, "Tree"=21819, "Tree 1"=21793, "Trigger"=1988, "TriggerList"=1989, "Two Button Dialog"=1341, "Type Cast"=1166, "Type and Creator"=1434, "UDP Close"=1726, "UDP Multicast Open"=1727, "UDP Network Connection Refnum"=3418, "UDP Open"=1723, "UDP Read"=1724, "UDP Write"=1725, "UTF-8 to Text"=23067, "Unbitpack from Array"=3136, "Unbundle"=2048, "Unbundle By Name"=2058, "Unflatten From String"=1165, "Unflatten From XML"=8401, "Unleak Variant Value Reference"=2411, "Unpackage Matrix"=23000, "Unregister For Events"=2076, "Unregister Session"=2320, "Up Arrow"=3823, "Up Bow Valve"=3703, "Up Bow Valve 1"=3803, "Up Bow Valve 2"=21763, "Up Rect Valve"=3702, "Up Rect Valve 1"=21762, "Up Rect Valve 2"=3802, "Up Tee"=3712, "Up Tee 1"=3812, "User Defined Refnum"=3428, "User Defined Refnum Tag"=21745, "User Defined Refnum Tag 1"=3429, "User Defined Refnum Tag Constant"=3426, "User Defined Refnum Tag Flatten"=21747, "User Defined Refnum Tag Flatten 1"=3454, "User Defined Tag"=21749, "User Defined Tag 1"=3329, "User Defined Tag Constant"=2114, "User Item"=3506, "VI Library"=1425, "VI Refnum"=3422, "VI Server Reference"=2091, "VISA Assert Interrupt Signal"=2309, "VISA Assert Trigger"=1929, "VISA Assert Utility Signal"=2310, "VISA Clear"=1927, "VISA Close"=1922, "VISA Disable Event"=1940, "VISA Discard Events"=1941, "VISA Enable Event"=1942, "VISA Find Resource"=1923, "VISA Flush I/O Buffer"=2302, "VISA GPIB Command"=2315, "VISA GPIB Control ATN"=2316, "VISA GPIB Control REN"=2304, "VISA GPIB Pass Control"=2317, "VISA GPIB Send IFC"=2318, "VISA In 16"=1930, "VISA In 32"=1944, "VISA In 64"=2140, "VISA In 8"=1936, "VISA Lock"=1993, "VISA Map Address"=1932, "VISA Map Trigger"=2311, "VISA Memory Allocation"=1997, "VISA Memory Allocation Ex"=2146, "VISA Memory Free"=1998, "VISA Move"=2303, "VISA Move In 16"=1948, "VISA Move In 32"=1991, "VISA Move In 64"=2144, "VISA Move In 8"=1946, "VISA Move Out 16"=1949, "VISA Move Out 32"=1992, "VISA Move Out 64"=2145, "VISA Move Out 8"=1947, "VISA Open"=2308, "VISA Out 16"=1931, "VISA Out 32"=1945, "VISA Out 64"=2141, "VISA Out 8"=1937, "VISA Peek 16"=1934, "VISA Peek 32"=1995, "VISA Peek 64"=2142, "VISA Peek 8"=1938, "VISA Poke 16"=1935, "VISA Poke 32"=1996, "VISA Poke 64"=2143, "VISA Poke 8"=1939, "VISA Read"=1925, "VISA Read STB"=1928, "VISA Read To File"=2313, "VISA Refnum to Session"=2300, "VISA Resource Name"=3421, "VISA Set I/O Buffer Size"=2301, "VISA Status Description"=1924, "VISA USB Control In"=2086, "VISA USB Control Out"=2087, "VISA Unlock"=1994, "VISA Unmap Address"=1933, "VISA Unmap Trigger"=2312, "VISA VXI Cmd or Query"=2305, "VISA Wait on Event"=1943, "VISA Write"=1926, "VISA Write From File"=2314, "VISA resource name"=3409, "VISA resource name 1"=21737, "Variable Class Specifier Constant"=2106, "Variable Configuration"=3475, "Variant"=3310, "Variant To Data"=8003, "Variant To Flattened String"=8203, "Vert Line"=3822, "Vert Pipe"=3816, "Vert Pipe 1"=3716, "Vert Rocker"=21740, "Vertical Fill Slide"=21014, "Vertical Fill Slide 1"=3009, "Vertical Graduated Bar"=21107, "Vertical Pointer Slide"=21017, "Vertical Pointer Slide 1"=3007, "Vertical Progress Bar"=21104, "Vertical Scrollbar"=21111, "Vertical Slide"=3004, "Vertical Slide Switch"=21741, "Vertical Slide Switch 1"=3115, "Vertical Smooth Box"=3634, "Vertical Splitter Bar"=21860, "Vertical Splitter Bar (Classic)"=21862, "Vertical Splitter Bar (System)"=21864, "Vertical Switch"=3109, "Vertical Toggle Switch"=21005, "Vertical Toggle Switch 1"=3111, "Volume Info"=1414, "Wait (ms)"=1302, "Wait For Activity"=1722, "Wait For Front Panel Activity"=1328, "Wait Until Next ms Multiple"=1327, "Wait for GPIB RQS"=1952, "Wait on Notification"=9105, "Wait on Notification from Multiple"=9106, "Wait on Notification from Multiple with Notifier History"=9132, "Wait on Notification with Notifier History"=9131, "Wait on Occurrence"=1701, "WaitSRQ"=1990, "Waveform Chart"=21010, "Waveform Chart 1"=3501, "Waveform Chart 2"=21717, "Waveform Graph"=21703, "Waveform Graph 1"=3504, "While Loop"=2003, "While Loop 1"=2352, "White Space?"=1125, "Write Datalog"=8079, "Write Device"=1431, "Write File"=1408, "Write Variable"=23782, "Write to Binary File"=8078, "Write to Text File"=8080, "XY Graph"=21716, "XY Graph 1"=3500, "Y-th Root of X"=23062]
                # "Get All Source\n(Right Terminals)"
                # "Get All nodes Drain Term Sources and get these Source Nodes\nAll drina terms.\nRemove the Drains terms that exists in the Nodes\nWe have in the array.\n==> Now we have some Source Nodes and their\nDrain Terminals that should be rewired are we're done"
                # "Last GetAtt ErrorOut"
                # "Last GetAtt ErrorOut"
                # "SetAtt Att Input Term"
                # "We need to add all nodes(SubVIs) between ErrorOut on last Get\nto the Error In of the SetAtt"
                # "Delete Wires to nodes"
                # "GetAtt No 1"
                # "GetAttToModifyForOtherlcassesIfNeeded"
                # "SetMod-VI"
                # "Rewire all nodes\nIf node when to GetAtt wire to DVR Inout Term\nIf node went to SetAtt wrie to DVR Out"
                # "DVR Ref"
                # "Remove Nodes that can be outside IPE"
                # "Get only Node Nodes"
                n44 = for {
                  tunnel: w220 -> [w587] mode=indexing
                  shift-right: [w574] -> w213
                  shift-left: w148 -> [w584]
                  tunnel: w146 -> [w578]
                  tunnel: w218 -> [w577]
                  tunnel: w217 -> [w576]
                  tunnel: w216 -> [w575]
                  shift-right: [w573] -> w214
                  shift-left: w193 -> [w572]
                  shift-right: [w571] -> w212
                  shift-left: w193 -> [w570]
                  shift-right: [w568] -> w206
                  shift-left: w193 -> [w569]
                  shift-right: [w566] -> w192
                  shift-left: w193 -> [w567]
                  tunnel: w191 -> [w565]
                  shift-right: [w564] -> w153
                  shift-left: w155 -> [w563]
                  # "GetAttSubVI"
                  n45 = To More Specific Class(target class=refnum<vi> refnum ("WhileLoop"), reference=w587, error in=w584) -> (specific class reference=w586:refnum<vi>, error out=w585:errorcluster)
                  n46 = property class="SubVI"(reference=w586, error in=w585) -> (reference out=w583:refnum<vi>, error out=w582:errorcluster, "VIName"=w581:string)
                  n47 = Match Pattern(string=w581, regular expression=w565) -> (offset past match=w580:i32)  [unwired: 1 in, 3 out]
                  n48 = Greater Or Equal To 0?(x=w580) -> (x >= 0?=w579:bool)
                  n49 = case shown="True" w579 {
                    tunnel: w583 -> [_ w614]
                    tunnel: w582 -> [w594 w613]
                    tunnel: w578 -> [_ w612]
                    tunnel: w577 -> [_ w611]
                    tunnel: w576 -> [_ w610]
                    tunnel: w575 -> [_ w609]
                    tunnel: [w594 w608] -> w574
                    tunnel: [w593 w607] -> w573
                    tunnel: w572 -> [w593 w606]
                    tunnel: [w592 w603] -> w571
                    tunnel: w570 -> [w592 w604]
                    tunnel: [w591 w601] -> w568
                    tunnel: w569 -> [w591 w600]
                    tunnel: [w590 w598] -> w566
                    tunnel: w567 -> [w590 w597]
                    tunnel: [w589 w595] -> w564
                    tunnel: w563 -> [w589 _]
                    frame False {
                    }
                    frame True {
                      n50 = property class="SubVI"(reference=w614, error in=w613) -> (reference out=w595:refnum<vi>, error out=w608:errorcluster, "Terms[]"=w605:refnum<vi>[])
                      n51 = Index Array(array=w605, index #1=w612, index #2=w611, index #3=w610, index #4=w609) -> (element #1=w596:refnum<vi>, element #2=w602:refnum<vi>, element #4=w599:refnum<vi>)  [unwired: 1 out]
                      n52 = Build Array (concatenate)(w606, w605) -> (w607:refnum<vi>[])
                      n53 = Build Array (concatenate)(w597, w596) -> (w598:refnum<vi>[])
                      n54 = Build Array (concatenate)(w604, w602) -> (w603:refnum<vi>[])
                      n55 = Build Array (concatenate)(w600, w599) -> (w601:refnum<vi>[])
                    }
                  }
                }
                n56 = To More Specific Class(target class=refnum<vi> refnum ("element"), reference=w237, error in=w213) -> (specific class reference=w177:refnum<vi>, error out=w231:errorcluster)
                n57 = property class="SubVI"(reference=w153) -> ("Terms[]"=w152:refnum<vi>[])  [unwired: 1 in, 2 out]
                n58 = for {
                  tunnel: w152 -> [w253] mode=indexing
                  shift-right: [w250] -> w151
                  shift-left: refnum<vi>[] [] -> [w251]
                  n59 = property class="Term"(reference=w253) -> (reference out=w252:refnum<vi>, "IsSource"=w249:bool, "Wire"=w246:refnum<vi>)  [unwired: 1 in, 1 out]
                  n60 = Not A Number/Path/Refnum?(number/path/refnum=w246) -> (NaN/Path/Refnum?=w248:bool)
                  n61 = Compound Arithmetic op=AND(w249, invert w248) -> (w247:bool)
                  n62 = case shown="False" w247 {
                    tunnel: w252 -> [w254 w258]
                    tunnel: w251 -> [w255 w257]
                    tunnel: [w255 w256] -> w250
                    frame False {
                      n63 = Close Reference(reference=w254) -> ()  [unwired: 1 in, 1 out]
                    }
                    frame True {
                      n64 = Build Array (concatenate)(w257, w258) -> (w256:refnum<vi>[])
                    }
                  }
                  n65 = Close Reference(reference=w246) -> ()  [unwired: 1 in, 1 out]
                }
                n66 = property class="SubVI"(reference=w177, error in=w231) -> (error out=w226:errorcluster, "Terms[]"=w215:refnum<vi>[])  [unwired: 1 out]
                n67 = call <resource>:"Scripting_SortTerminals.vi"("Terminals[]"=w215) -> ("TerminalsOut[]"=w224:refnum<vi>[])  [unwired: 8 in, 2 out]
                n68 = Build Array (concatenate)(w208, w206) -> (w207:refnum<vi>[])
                n69 = Index Array(array=w224, index=w223) -> (element=w160:refnum<vi>)
                n70 = Delete From Array(array=w192) -> (deleted portion=w180:refnum<vi>)  [unwired: 2 in, 1 out]
                n71 = Build Array (concatenate)(w219, w212) -> (w161:refnum<vi>[])
                n72 = for {
                  tunnel: [w526] -> w227 mode=indexing
                  tunnel: [w528] -> w221 mode=indexing
                  tunnel: w161 -> [w529] mode=indexing
                  shift-right: [w531] -> w225
                  shift-left: w226 -> [w532]
                  tunnel: [w525] -> w211 mode=indexing
                  tunnel: w160 -> [w523]
                  tunnel: T1 {"ReachedANyOfTheseNodes"=[], "NodeType"=[], "VINames"=["SetClassModifiedAttributes.vi$", "SetModifiedAttributes.vi$", "GetClassAttributes.vi$", "GetAttributes.vi$", "SetModifiedAttributes.vi$", "SetModifiedClassAttributes.vi$"], "AddTheseNodes"=FALSE, "ALsoSerachOtherDrainNodes"=FALSE} ("StopCriteria") -> [w514]
                  tunnel: w151 -> [_]
                  n73 = call <resource>:"Scripting_FollowWireDownStreams.vi"("Term Refnum"=w529, "NodeTypesToFind"=string[] ["NamedUnbundler", "NamedBundler"], "error in"=w532, "MainitainDataType"=TRUE ("MainitainDateType(True)"), "StopCriteria"=T1 {"ReachedANyOfTheseNodes"=[], "NodeType"=["SubVI", "PolymorphicSubVI", "CallParentNode", "DynamicDispatchSubVI"], "VINames"=[], "AddTheseNodes"=FALSE, "ALsoSerachOtherDrainNodes"=FALSE}) -> ("Nodes"=w519:refnum<vi>[], "NodeTypes"=w522:string[], "error out"=w533:errorcluster)  [unwired: 11 in, 1 out]
                  n74 = Reverse 1D Array(array=w522) -> (reversed array=w521:string[])
                  n75 = call <resource>:"Scripting_GetAllNodesConnectedToTerminal.vi"("Term Refnum"=w529, "error in"=w533, "StopCriteria"=w514) -> ("Nodes"=w535:refnum<vi>[], "error out"=w534:errorcluster)  [unwired: 13 in, 2 out]
                  n76 = Search 1D Array(1D array=w521, element="NamedBundler" ("regular expression")) -> (index of element=w517:i32)  [unwired: 1 in]
                  n77 = Reverse 1D Array(array=w519) -> (reversed array=w518:refnum<vi>[])
                  n78 = Index Array(array=w518, index=w517) -> (element=w516:refnum<vi>)
                  n79 = for {
                    tunnel: w535 -> [w538] mode=indexing
                    shift-right: [w543] -> w531
                    shift-left: w534 -> [w545]
                    shift-right: [w546] -> w527
                    shift-left: T3[] [] -> [w547]
                    tunnel: w523 -> [w540]
                    tunnel: w516 -> [w539]
                    n80 = call <resource>:"Scripting_GetNodeInfo.vi"("Node Refnum Or Constrol/Indicator/Constant"=w538, "error in (no error)"=w545) -> ("OK"=w544:bool, "NodeInfo"=w542:T3, "error out"=w543:errorcluster)  [unwired: 15 in]
                    n81 = Equal?(x=w538, y=w539) -> (x = y?=w537:bool)
                    n82 = case shown="True" w537 {
                      tunnel: w542 -> [w556 w558]
                      tunnel: [w557 w558] -> w541
                      tunnel: w540 -> [w548 _]
                      frame True {
                        w554 = 0 ("index")
                        n83 = Unbundle By Name(w556) -> ("SourcesDrainTerms"=w555:cluster{"DrainsTerms":refnum<vi>[]}[])
                        n84 = Index Array(array=w555, index=w554) -> (element=w552:cluster{"DrainsTerms":refnum<vi>[]})
                        n85 = Unbundle(w552) -> ("DrainsTerms"=w551:refnum<vi>[])
                        n86 = Build Array (concatenate)(w551, w548) -> (w550:refnum<vi>[])
                        n87 = Bundle(w550) -> (w549:cluster{refnum<vi>[]})  [unwired: 1 in]
                        n88 = Replace Array Subset(array=w555, new element=w549, index=w554) -> (w553:cluster{"DrainsTerms":refnum<vi>[]}[])
                        n89 = Bundle By Name(cluster=w556, "SourcesDrainTerms"=w553) -> (w557:T3)
                      }
                      frame False {
                      }
                    }
                    n90 = case shown="False" w544 {
                      tunnel: w547 -> [w559 w562]
                      tunnel: [w559 w561] -> w546
                      tunnel: w541 -> [_ w560]
                      frame False {
                      }
                      frame True {
                        n91 = Build Array (concatenate)(w562, w560) -> (w561:T3[])
                      }
                    }
                  }
                  n92 = Bundle("Nodes"=w519) -> (w525:cluster{"Nodes":refnum<vi>[]})  [unwired: 1 in]
                  n93 = Bundle("NodeTypes"=w522) -> (w528:cluster{"NodeTypes":string[]})  [unwired: 1 in]
                  n94 = Bundle(w527) -> (w526:cluster{T3[]})  [unwired: 1 in]
                }
                n95 = property class="Term"(reference=w180) -> ("Wire.Terms[]"=w178:refnum<vi>[])  [unwired: 1 in, 2 out]
                n96 = Search 1D Array(1D array=w178, element=w180) -> (index of element=w179:i32)  [unwired: 1 in]
                n97 = Delete From Array(array=w178, index=w179) -> ()  [unwired: 1 in, 2 out]
                n98 = call <resource>:"ConvertGoop3ToGoop4_SelectNodesToBeInsideIP.vi"("NodesIn"=w227, "BundleNodes"=w211, "BundleNodeTypes"=w221, "error in"=w225, "GetAttribute_AttributeTerminal"=w161, "FirstGetAttributesDrainsTerminals"=w156, "LastGetAttributesSourceTerminals"=w151) -> ("NodesOut"=w166:cluster{"NodesIn":T3[]}[], "IPE-Position"=w173:T4, "IPE-Frame Size"=w172:T5, "error out"=w171:errorcluster)  [unwired: 5 in]
                n99 = for {
                  tunnel: w166 -> [w284] mode=indexing
                  shift-right: [w285] -> w169
                  shift-left: refnum<vi>[] [] -> [w286]
                  n100 = Unbundle(w284) -> ("NodesIn"=w283:T3[])
                  n101 = for {
                    tunnel: w283 -> [w290] mode=indexing
                    shift-right: [w287] -> w285
                    shift-left: w286 -> [w288]
                    n102 = Unbundle By Name(w290) -> ("Drains"=w289:refnum<vi>[])
                    n103 = for {
                      tunnel: w289 -> [w292] mode=indexing
                      shift-right: [w291] -> w287
                      shift-left: w288 -> [w293]
                      n104 = Build Array (concatenate)(w293, w292) -> (w291:refnum<vi>[])
                    }
                  }
                }
                n105 = for {
                  tunnel: w166 -> [w298] mode=indexing
                  shift-right: [w299] -> w170
                  shift-left: w171 -> [w300]
                  tunnel: w169 -> [w296]
                  shift-right: [w294] -> w167
                  shift-left: T2 [] -> [w295]
                  n106 = Unbundle(w298) -> ("NodesIn"=w297:T3[])
                  n107 = for {
                    tunnel: w297 -> [w309] mode=indexing
                    shift-right: [w306] -> w299
                    shift-left: w300 -> [w307]
                    tunnel: w296 -> [w305]
                    shift-right: [w303] -> w294
                    shift-left: w295 -> [w301]
                    n108 = Unbundle By Name(w309) -> ("DrainsSourcesTerms"=w308:refnum<vi>[])  [unwired: 1 out]
                    n109 = for {
                      tunnel: w308 -> [w313] mode=indexing
                      shift-right: [w314] -> w306
                      shift-left: w307 -> [w316]
                      tunnel: w305 -> [w315]
                      shift-right: [w310] -> w304
                      shift-left: T2 [] -> [w311]
                      n110 = Not A Number/Path/Refnum?(number/path/refnum=w313) -> (NaN/Path/Refnum?=w312:bool)
                      n111 = case shown="False" w312 {
                        tunnel: w316 -> [w328 w339]
                        tunnel: w315 -> [w326 _]
                        tunnel: [w322 w339] -> w314
                        tunnel: w313 -> [w320 _]
                        tunnel: w311 -> [w318 w340]
                        tunnel: [w319 w340] -> w310
                        frame False {
                          n112 = call <resource>:"Scripting_GetTerminalWireConnectionPoints.vi"("Term Refnum In"=w320, "error in"=w328) -> ("Term Refnum Out"=w323:refnum<vi>, "WireTermSource"=w321:refnum<vi>, "AllWireTerminalDrains"=w327:refnum<vi>[], "error out"=w322:errorcluster)  [unwired: 9 in, 5 out]
                          n113 = Close Reference(reference=w321) -> ()  [unwired: 1 in, 1 out]
                          n114 = for {
                            tunnel: w327 -> [w331] mode=indexing
                            tunnel: w326 -> [w333]
                            shift-right: [w329] -> w324
                            shift-left: refnum<vi>[] [] -> [w330]
                            n115 = Search 1D Array(1D array=w333, element=w331) -> (index of element=w332:i32)  [unwired: 1 in]
                            n116 = case shown="0, Default" w332 {
                              tunnel: w331 -> [w335 w336]
                              tunnel: w330 -> [w334 w337]
                              tunnel: [w334 w338] -> w329
                              frame 0, Default {
                                n117 = Close Reference(reference=w335) -> ()  [unwired: 1 in, 1 out]
                              }
                              frame -1 {
                                n118 = Build Array (concatenate)(w337, w336) -> (w338:refnum<vi>[])
                              }
                            }
                          }
                          n119 = Bundle("Term Refnum Out"=w323, w324) -> (w317:T6)  [unwired: 1 in]
                          n120 = Build Array (concatenate)(w318, w317) -> (w319:T2)
                        }
                        frame True {
                        }
                      }
                    }
                    n121 = Build Array (concatenate)(w301, w304) -> (w303:T2)
                  }
                }
                n122 = for {
                  tunnel: w166 -> [w491] mode=indexing
                  shift-right: [w492] -> w222
                  shift-left: w170 -> [w493]
                  n123 = Unbundle(w491) -> ("NodesIn"=w490:T3[])
                  n124 = for {
                    tunnel: w490 -> [w497] mode=indexing
                    shift-right: [w494] -> w492
                    shift-left: w493 -> [w495]
                    n125 = Unbundle By Name(w497) -> ("Terms"=w496:refnum<vi>[])
                    n126 = for {
                      tunnel: w496 -> [w501] mode=indexing
                      shift-right: [w498] -> w494
                      shift-left: w495 -> [w502]
                      n127 = Not A Number/Path/Refnum?(number/path/refnum=w501) -> (NaN/Path/Refnum?=w500:bool)
                      n128 = case shown="False" w500 {
                        tunnel: w502 -> [w508 w513]
                        tunnel: [w505 w513] -> w499
                        tunnel: w501 -> [w503 _]
                        frame False {
                          n129 = property class="Term"(reference=w503, error in=w508) -> (error out=w507:errorcluster, "Wire"=w504:refnum<vi>)  [unwired: 1 out]
                          n130 = Not A Number/Path/Refnum?(number/path/refnum=w504) -> (NaN/Path/Refnum?=w506:bool)
                          n131 = case shown="False" w506 {
                            tunnel: w504 -> [w511 _]
                            tunnel: w507 -> [w510 w512]
                            tunnel: [w509 w512] -> w505
                            frame False {
                              n132 = invoke class="Wire" method="Delete"(reference=w511, error in=w510) -> (error out=w509:errorcluster)  [unwired: 1 in, 2 out]
                            }
                            frame True {
                            }
                          }
                        }
                        frame True {
                        }
                      }
                      n133 = call <vilib>:"Clear Errors.vi"("error in (no error)"=w499) -> ("error out"=w498:errorcluster)  [unwired: 6 in]
                    }
                  }
                }
                n134 = New VI Object(vi object class=w234, owner refnum=w230, style=w235, position/next to=w173, 8:w222) -> (object refnum=w233:refnum<vi>, 0:w232:errorcluster)  [unwired: 3 in]
                n135 = property class="InPlaceStruct"(reference=w233, error in=w232, "Frame Size"=w172, "Position"=w173, "AutoSize"=TRUE ("AutoSize To Fit Contents?")) -> (reference out=w203:refnum<vi>, error out=w229:errorcluster)
                n136 = for {
                  tunnel: w203 -> [w392]
                  tunnel: [w387] -> w205 mode=indexing
                  tunnel: [w373] -> w159 mode=indexing
                  tunnel: w207 -> [w385] mode=indexing
                  shift-right: [w381] -> _
                  shift-left: u32 24 ("Y Position") -> [w379]
                  shift-right: [w372] -> w204
                  shift-left: w229 -> [w391]
                  # "Wire Nodes Up"
                  n137 = invoke class="InPlaceStruct" method="Add In Place Pair"(reference=w392, error in=w391, "Y Position"=w379, "DPID"=u32 339) -> (error out=w382:errorcluster, "Add In Place Pair"=w390:refnum<vi>)  [unwired: 1 in, 3 out]
                  n138 = Add(x=w379, y=u32 32) -> (x+y=w381:u32)
                  n139 = property class="InPlaceBorderNode"(reference=w390, error in=w382) -> (reference out=w388:refnum<vi>, error out=w383:errorcluster, "Terms[]"=w389:refnum<vi>[], "Partner"=w386:refnum<vi>)
                  n140 = Index Array(array=w389) -> (element #1=w375:refnum<vi>, element #2=w387:refnum<vi>, element #3=w377:refnum<vi>)  [unwired: 3 in]
                  n141 = call <resource>:"Scripting_WireTerminals.vi"("error in"=w383, "Term 2"=w375, "Term 1"=w385) -> ("error out"=w384:errorcluster)  [unwired: 8 in]
                  n142 = property class="InPlaceBorderNode"(reference=w386, error in=w384) -> (reference out=w378:refnum<vi>, error out=w376:errorcluster, "Terms[]"=w374:refnum<vi>[])
                  n143 = Close Reference(reference=w375, error in (no error)=w376) -> ()  [unwired: 1 out]
                  n144 = Close Reference(reference=w377, error in (no error)=w376) -> ()  [unwired: 1 out]
                  n145 = Delete From Array(array=w374, index=0) -> (deleted portion=w373:refnum<vi>, array with subset deleted=w371:refnum<vi>[])  [unwired: 1 in]
                  n146 = Close Reference(reference=w378, error in (no error)=w376) -> (error out=w372:errorcluster)
                  n147 = Close Reference(reference=w388, error in (no error)=w376) -> ()  [unwired: 1 out]
                  n148 = Close Reference(reference=w371) -> ()  [unwired: 1 in, 1 out]
                }
                n149 = for {
                  tunnel: w203 -> [w478]
                  tunnel: w166 -> [w475] mode=indexing
                  tunnel: w173 -> [w476]
                  shift-right: [w477] -> w210
                  shift-left: w204 -> [w479]
                  n150 = Unbundle(w475) -> ("NodesIn"=w474:T3[])
                  n151 = for {
                    tunnel: w478 -> [w489]
                    tunnel: w474 -> [w488] mode=indexing
                    tunnel: w476 -> [w486]
                    shift-right: [w484] -> w477
                    shift-left: w479 -> [w485]
                    n152 = Unbundle By Name(w488) -> ("ObjectRef"=w480:refnum<vi>, "UpperLeftPosition"=w487:cluster{"Left":i32, "Top":i32})
                    n153 = Subtract(x=w487, y=w486) -> (x-y=w482:T4)
                    n154 = Subtract(x=w482, y=cluster{dbl, dbl} {4.0, 4.0}) -> (x-y=w481:cluster{dbl, dbl})
                    n155 = invoke class="GObj" method="Move"(reference=w480, error in=w485, "position"=w481, "owner"=w489) -> (error out=w484:errorcluster)  [unwired: 2 in, 5 out]
                  }
                }
                n156 = for {
                  tunnel: w205 -> [w403]
                  tunnel: w160 -> [w402]
                  tunnel: w159 -> [w401] mode=indexing
                  tunnel: w166 -> [w397] mode=indexing
                  tunnel: w161 -> [w399]
                  shift-right: [w398] -> w163
                  shift-left: w210 -> [w400]
                  shift-right: [w394] -> _
                  shift-left: cluster{"Term":refnum<vi>, "Term":refnum<vi>}[] [] -> [w395]
                  n157 = Unbundle(w397) -> ("NodesIn"=w396:T3[])
                  n158 = for {
                    shift-right: [w409] -> w398
                    shift-left: w400 -> [w414]
                    tunnel: w396 -> [w418] mode=indexing
                    tunnel: w399 -> [w413]
                    tunnel: w403 -> [w415]
                    tunnel: w402 -> [w408]
                    tunnel: w401 -> [w407]
                    shift-right: [w404] -> w394
                    shift-left: w395 -> [w405]
                    n159 = Unbundle By Name(w418) -> ("Sources"=w412:refnum<vi>[], "Drains"=w417:refnum<vi>[], "DrainsSourcesTerms"=w416:refnum<vi>[], "SourcesDrainTerms"=w411:cluster{"DrainsTerms":refnum<vi>[]}[])
                    n160 = for {
                      tunnel: w417 -> [w449] mode=indexing
                      tunnel: w416 -> [w455] mode=indexing
                      tunnel: w413 -> [w458]
                      tunnel: w415 -> [w456]
                      shift-right: [w459] -> w410
                      shift-left: w414 -> [w460]
                      shift-right: [w454] -> w406
                      shift-left: w405 -> [w453]
                      n161 = Search 1D Array(1D array=w458, element=w455) -> (index of element=w457:i32)  [unwired: 1 in]
                      n162 = case shown="-1" w457 {
                        selector: w457 -> [w472 _]
                        tunnel: w456 -> [w471 _]
                        tunnel: [w470 w473] -> w450
                        tunnel: w455 -> [_ w473]
                        frame Default {
                          n163 = Index Array(array=w471, index=w472) -> (element=w470:refnum<vi>)
                        }
                        frame -1 {
                        }
                      }
                      n164 = Bundle("Term"=w450, "Term"=w449) -> (w451:cluster{"Term":refnum<vi>, "Term":refnum<vi>})  [unwired: 1 in]
                      n165 = Search 1D Array(1D array=w453, element=w451) -> (index of element=w452:i32)  [unwired: 1 in]
                      n166 = case shown="-1" w452 {
                        tunnel: w460 -> [w462 w469]
                        tunnel: [w462 w468] -> w459
                        tunnel: w449 -> [_ w467]
                        tunnel: w450 -> [_ w466]
                        tunnel: w453 -> [w461 w465]
                        tunnel: [w461 w464] -> w454
                        tunnel: w451 -> [_ w463]
                        frame 0, Default {
                        }
                        frame -1 {
                          n167 = Build Array (concatenate)(w465, w463) -> (w464:cluster{"Term":refnum<vi>, "Term":refnum<vi>}[])
                          n168 = call <resource>:"Scripting_WireTerminals.vi"("error in"=w469, "Term 2"=w467, "Term 1"=w466) -> ("error out"=w468:errorcluster)  [unwired: 8 in]
                        }
                      }
                    }
                    n169 = for {
                      tunnel: w412 -> [w427] mode=indexing
                      tunnel: w411 -> [w425] mode=indexing
                      tunnel: w408 -> [w426]
                      tunnel: w407 -> [w424]
                      shift-right: [w422] -> w409
                      shift-left: w410 -> [w423]
                      shift-right: [w420] -> w404
                      shift-left: w406 -> [w419]
                      n170 = Unbundle(w425) -> ("DrainsTerms"=w421:refnum<vi>[])
                      n171 = for {
                        tunnel: w427 -> [w430]
                        tunnel: w426 -> [w439]
                        tunnel: w424 -> [w437]
                        tunnel: w421 -> [w436] mode=indexing
                        shift-right: [w433] -> w422
                        shift-left: w423 -> [w428]
                        shift-right: [w432] -> w420
                        shift-left: w419 -> [w431]
                        n172 = Not Equal?(x=w436, y=w439) -> (x != y?=w438:bool)
                        n173 = Select(t=w436, s=w438, f=w437) -> (s? t:f=w429:refnum<vi>)
                        n174 = Bundle("Term"=w430, "Term"=w429) -> (w435:cluster{"Term":refnum<vi>, "Term":refnum<vi>})  [unwired: 1 in]
                        n175 = Search 1D Array(1D array=w431, element=w435) -> (index of element=w434:i32)  [unwired: 1 in]
                        n176 = case shown="-1" w434 {
                          tunnel: w428 -> [w441 w448]
                          tunnel: [w441 w447] -> w433
                          tunnel: w429 -> [_ w446]
                          tunnel: w430 -> [_ w445]
                          tunnel: w431 -> [w440 w444]
                          tunnel: [w440 w443] -> w432
                          tunnel: w435 -> [_ w442]
                          frame 0, Default {
                          }
                          frame -1 {
                            n177 = Build Array (concatenate)(w444, w442) -> (w443:cluster{"Term":refnum<vi>, "Term":refnum<vi>}[])
                            n178 = call <resource>:"Scripting_WireTerminals.vi"("error in"=w448, "Term 2"=w446, "Term 1"=w445) -> ("error out"=w447:errorcluster)  [unwired: 8 in]
                          }
                        }
                      }
                    }
                  }
                }
                n179 = Close Reference(reference=w205, error in (no error)=w163) -> ()  [unwired: 1 out]
                n180 = for {
                  tunnel: w167 -> [w274] mode=indexing
                  shift-right: [w275] -> w162
                  shift-left: w163 -> [w276]
                  n181 = Unbundle(w274) -> ("Term Refnum Out"=w278:refnum<vi>, w277:refnum<vi>[])
                  n182 = for {
                    tunnel: w278 -> [w282]
                    tunnel: w277 -> [w281] mode=indexing
                    shift-right: [w279] -> w275
                    shift-left: w276 -> [w280]
                    n183 = call <resource>:"Scripting_WireTerminals.vi"("error in"=w280, "Term 2"=w281, "Term 1"=w282) -> ("error out"=w279:errorcluster)  [unwired: 8 in]
                  }
                }
                n184 = disable-structure shown="Enabled" {
                  disable-tunnel: w165 -> [w368 _]
                  disable-tunnel: w203 -> [w365 _]
                  disable-tunnel: w162 -> [w361 w369]
                  disable-tunnel: [w357 w369] -> w202
                  disable-tunnel: [w357 w369] -> w197
                  frame Enabled {
                    n185 = property class="VI"(reference=w368, error in=w361) -> (error out=w362:errorcluster, "Diagram"=w355:refnum<vi>)  [unwired: 1 out]
                    n186 = invoke class="TopLvlDiag" method="Clear Selection"(reference=w355, error in=w362) -> (reference out=w367:refnum<vi>, error out=w363:errorcluster)  [unwired: 1 in, 1 out]
                    n187 = Build Array(w365) -> (w366:refnum<vi>[])
                    n188 = invoke class="TopLvlDiag" method="Make Selection"(reference=w367, error in=w363, "Objects"=w366) -> (reference out=w356:refnum<vi>, error out=w364:errorcluster)  [unwired: 1 in, 2 out]
                    n189 = invoke class="TopLvlDiag" method="CleanUp"(reference=w356, error in=w364) -> (reference out=w354:refnum<vi>, error out=w360:errorcluster)  [unwired: 2 in, 2 out]
                    n190 = invoke class="TopLvlDiag" method="Clear Selection"(reference=w354, error in=w360) -> (reference out=w359:refnum<vi>, error out=w358:errorcluster)  [unwired: 1 in, 1 out]
                    n191 = Close Reference(reference=w359, error in (no error)=w358) -> (error out=w357:errorcluster)
                  }
                  frame Disabled {
                  }
                }
                n192 = property class="SubVI"(reference=w177, error in=w197) -> (reference out=w194:refnum<vi>, error out=w196:errorcluster, "Terms[]"=w181:refnum<vi>[])
                n193 = call <resource>:"Scripting_IndicateConnectorPaneCorners.vi"("Terminals[]"=w181) -> ("RightLower"=w198:i32, "LeftLower"=w199:i32, "RightTop"=w200:i32, "LeftTop"=w201:i32)  [unwired: 7 in]
                n194 = Index Array(array=w181, index #1=w201, index #2=w200, index #3=w199, index #4=w198) -> (element #1=w195:refnum<vi>, element #2=w190:refnum<vi>, element #3=w187:refnum<vi>, element #4=w186:refnum<vi>)
                n195 = property class="Term"(reference=w190) -> ("Wire"=w189:refnum<vi>)  [unwired: 1 in, 2 out]
                n196 = Not A Number/Path/Refnum?(number/path/refnum=w189) -> (NaN/Path/Refnum?=w184:bool)
                n197 = case shown="True" w184 {
                  tunnel: w196 -> [w350 w351]
                  tunnel: w195 -> [w349 w353]
                  tunnel: [w345 w351] -> w188
                  tunnel: w190 -> [w347 _]
                  tunnel: w189 -> [w346 _]
                  frame False {
                    n198 = call <resource>:"Scripting_WireTerminals.vi"("error in"=w350, "CleanUpWire(True)"=FALSE, "Term 2"=w347, "Term 1"=w349) -> ("error out"=w345:errorcluster)  [unwired: 7 in]
                    n199 = Close Reference(reference=w346) -> ()  [unwired: 1 in, 1 out]
                  }
                  frame True {
                    n200 = property class="Term"(reference=w353) -> ("Wire"=w352:refnum<vi>)  [unwired: 1 in, 2 out]
                    n201 = invoke class="Wire" method="Delete"(reference=w352) -> ()  [unwired: 2 in, 3 out]
                  }
                }
                n202 = call <resource>:"Scripting_WireTerminals.vi"("error in"=w188, "CleanUpWire(True)"=FALSE, "Term 2"=w186, "Term 1"=w187) -> ("error out"=w183:errorcluster)  [unwired: 7 in]
                n203 = invoke class="SubVI" method="Delete"(reference=w194, error in=w183) -> (error out=w182:errorcluster)  [unwired: 1 in, 2 out]
                n204 = case shown="False" w184 {
                  tunnel: w180 -> [w343 _]
                  tunnel: w182 -> [w342 w344]
                  tunnel: [w341 w344] -> w164
                  frame False {
                    n205 = call <resource>:"Scripting_CleanUpTermWire.vi"("error in"=w342, "TermIn"=w343) -> ("error out"=w341:errorcluster)  [unwired: 8 in, 1 out]
                  }
                  frame True {
                  }
                }
                n206 = Close Reference(reference=w181, error in (no error)=w182) -> ()  [unwired: 1 out]
                n207 = Build Array (concatenate)(w175, w177) -> (w176:refnum<vi>[])
                n208 = Close Reference(reference=w203, error in (no error)=w202) -> ()  [unwired: 1 out]
                n209 = stacked-sequence {
                  tunnel: w167 -> [w261]
                  tunnel: w166 -> [w259]
                  tunnel: w164 -> [w260]
                  tunnel: [w260] -> w150
                  frame #0 {
                    n210 = for {
                      tunnel: w261 -> [w273] mode=indexing
                      n211 = Unbundle(w273) -> ("Term Refnum Out"=w271:refnum<vi>, w272:refnum<vi>[])
                      n212 = Close Reference(reference=w272) -> ()  [unwired: 1 in, 1 out]
                      n213 = Close Reference(reference=w271) -> ()  [unwired: 1 in, 1 out]
                    }
                    n214 = for {
                      tunnel: w259 -> [w263] mode=indexing
                      n215 = Unbundle(w263) -> ("NodesIn"=w262:T3[])
                      n216 = for {
                        tunnel: w262 -> [w268] mode=indexing
                        n217 = Unbundle(w268) -> ("ObjectRef"=w267:refnum<vi>, "Terms"=w266:refnum<vi>[], "DrainsSourcesTerms"=w265:refnum<vi>[], "SourcesDrainTerms"=w264:cluster{"DrainsTerms":refnum<vi>[]}[])  [unwired: 6 out]
                        n218 = for {
                          tunnel: w264 -> [w270] mode=indexing
                          n219 = Unbundle(w270) -> ("DrainsTerms"=w269:refnum<vi>[])
                          n220 = Close Reference(reference=w269) -> ()  [unwired: 1 in, 1 out]
                        }
                        n221 = Close Reference(reference=w267) -> ()  [unwired: 1 in, 1 out]
                        n222 = Close Reference(reference=w266) -> ()  [unwired: 1 in, 1 out]
                        n223 = Close Reference(reference=w265) -> ()  [unwired: 1 in, 1 out]
                      }
                    }
                  }
                }
                n224 = case shown="Error" w150 {
                  selector: w150 -> [w243 w244]
                  tunnel: w149 -> [_ w245]
                  tunnel: [w243 w244] -> w143
                  frame No Error {
                  }
                  frame Error {
                    n225 = invoke class="VI" method="Revert VI"(reference=w245) -> ()  [unwired: 2 in, 3 out]
                  }
                }
                n226 = Index Array(array=w147, index=w146) -> (element=w145:refnum<vi>)
                n227 = property class="Term"(reference=w145, error in=w143) -> ("Wire"=w141:refnum<vi>)  [unwired: 2 out]
                n228 = Not A Number/Path/Refnum?(number/path/refnum=w141) -> (NaN/Path/Refnum?=w144:bool)
                n229 = case shown="False" w144 {
                  tunnel: w143 -> [w240 w242]
                  tunnel: [w240 w242] -> w142
                  tunnel: w141 -> [w241 _]
                  frame False {
                    n230 = invoke class="Wire" method="RemoveLooseEnds"(reference=w241) -> (reference out=w239:refnum<vi>, error out=w238:errorcluster)  [unwired: 2 in, 1 out]
                    n231 = Close Reference(reference=w239, error in (no error)=w238) -> ()  [unwired: 1 out]
                  }
                  frame True {
                  }
                }
              }
            }
            n232 = Close Reference(reference=w91) -> ()  [unwired: 1 in, 1 out]
            n233 = Close Reference(reference=w83, error in (no error)=w110) -> (error out=w92:errorcluster)
          }
          frame False {
          }
        }
        n234 = Close Reference(reference=w38) -> ()  [unwired: 1 in, 1 out]
        n235 = Close Reference(reference=w37) -> ()  [unwired: 1 in, 1 out]
        n236 = Close Reference(reference=w36) -> ()  [unwired: 1 in, 1 out]
        n237 = Close Reference(reference=w26) -> ()  [unwired: 1 in, 1 out]
        n238 = Close Reference(reference=w33) -> ()  [unwired: 1 in, 1 out]
      }
      n239 = Close Reference(reference=w15) -> ()  [unwired: 1 in, 1 out]
      n240 = disable-structure shown="Enabled" {
        disable-tunnel: w5 -> [w23 _]
        disable-tunnel: w8 -> [w22 w24]
        disable-tunnel: [w21 w24] -> w7
        frame Disabled {
          n241 = invoke class="VI" method="BD.Remove Bad Wires"(reference=w23, error in=w22) -> (error out=w21:errorcluster)  [unwired: 1 in, 2 out]
        }
        frame Enabled {
        }
      }
      n242 = Close Reference(reference=w10) -> ()  [unwired: 1 in, 1 out]
    }
    frame Error {
    }
  }
  "error out" <- w3
  "ViRefOut" <- "ViRefIn"
